vi "REFPROPdll.vi"(8 "error in (no error)":errorcluster, 11 "Inputs":T2) -> (0 "error out":errorcluster, 3 "Outputs":T1)   [LabVIEW 2021]
doc: "subroutine REFPROPdll(hFld, hIn, hOut, iUnits, iMass, iFlag, a, b, zm, Output, hUnits, iUCode, x, y, x3, q, ierr, herr, hFld_length, hIn_length, hOut_length, hUnits_length, herr_length)\n\nCalculate the properties identified in the hOut string for the inputs specified in the hIn string for the fluid or\nmixture given in the hFld string. The unit identifier for the properties should be passed in the iUnits variable (as described below). Compositions can be sent as mole fractions or mass fractions in the zm array depending on the value of iMass.\n\nSeveral items must be considered before using this routine. The most important is the speed of calculations. The original fortran code that called dedicated functions such as TPRHO, TPFLSH, PHFLSH, and so on (mostly given in FLSH_SUB.FOR) and the non-iterative functions such as THERM and TRNPRP requires very little (or none) string comparisons and are quite fast. Multiple string comparisons are made to determine the inputs and outputs the user has selected. Due to the limitation of Fortran in string parsing, this will cause a dramatic increase in the time required to make the calculations, such as two to three times as long as the dedicated functions. Thus the ease of use of this REFPROP subroutine versus the speed of calculation from the older routines must be considered before developing any application.\n\nINPUTS:\nhFld -- Fluid string. See below.\nhIn -- Input string of properties being sent to the routine.\nhOut -- Various flags are available to gain access to all other features of the REFPROP program.\niUnits -- The unit system to be used for the input and output properties (such as SI, English, etc.) See the details much further below for a complete description of the iUnits input value. NOTE: A mass based value for iUnits does not imply that the input and output compositions are on a mass basis, this is specified with the iMass variable.\niMass -- Specifies if the input composition is mole or mass based.\n0 Input compositions given in mole fractions, quality on a molar basis.\n1 Input compositions given in mass fractions, quality on a mass basis. For two-phase states, the values in x and will be returned on a mass basis if iMass=1. NOTE: If the fluid string sent to this routine contains the word “mass” at the end (and thus contains the composition as well as the names of the fluids), this will have preference over the value of iMass when converting those compositions from a mass to a molar basis.\niFlag -- Flag to specify if the routine SATSPLN should be called (where a value of 1 activates the call). (Eventually this variable may be used to send multiple flags combined in this flag)\na -- First input property as specified in the hIn variable\nb -- Second input property as specified in the hIn variable\nzm -- Composition on a mole or mass basis depending on the value sent in iMass (array of size ncmax=20).\n\nOUTPUTS:\nOutput -- Array of properties specified by the hOut string (array of size 200 dimensioned as double precision). The number -9999970 will be returned when errors occur, and the number -9999990 will be returned when nothing was calculated. Read the comments in the ALLPROPS routine to fully understand the contents of this array.\nhUnits -- The units for the first property in the Output array. Strings such as a fluid name may also be passed back in this position. To obtain the units for all of the properties sent to the string, call the ALLPROPS routine instead.\niUCode -- Unit code that represents the units of the first property in the Output array. See below for further details.\nx -- Composition of the liquid phase (array of mole fractions of size 20) for two-phase states on a mole or mass basis depending on the value of iMass.\ny -- Composition of the vapor phase (array of mole fractions of size 20) for two-phase states on a mole or mass basis depending on the value of iMass.\nx3 -- Reserved for returning the composition of a second liquid phase for LLE or VLLE.\nq -- Vapor quality on a mole or mass basis depending on the value of iMass. (See subroutine ABFLSH for the definitions of values returned for this variable). To obtain the molar quality regardless of iMass, send “qmole” as an input in hIn, and vice-versa for “qmass”.\nierr -- Error flag\nherr -- Error string (character*255)\nhFld_length -- length of variable hFld (default: 10000)\nhIn_length -- length of variable hIn (default: 255)\nhOut_length -- length of variable hOut (default: 255)\nhUnits_length -- length of variable hUnits (default: 255)\nherr_length -- length of variable herr (default: 255)"
uses:
  REFPROP.dll
panel:
  # "REFPROP-REFPROPdll.vi"
  # "void REFPROPdll(char *hFld, char *hIn, char *hOut, int *iUnits, int *iMass, int *iFlag, double *a, double *b, double *z/* 20 */, double *Output/* 200 */, char *hUnits, int *iUCode, double *x/* 20 */, double *y/* 20 */, double *x3/* 20 */, double *q, int *ierr, char *herr, int hFld_length/* 10000 */, int hIn_length/* 255 */, int hOut_length/* 255 */, int hUnits_length/* 255 */, int herr_length/* 255 */);"
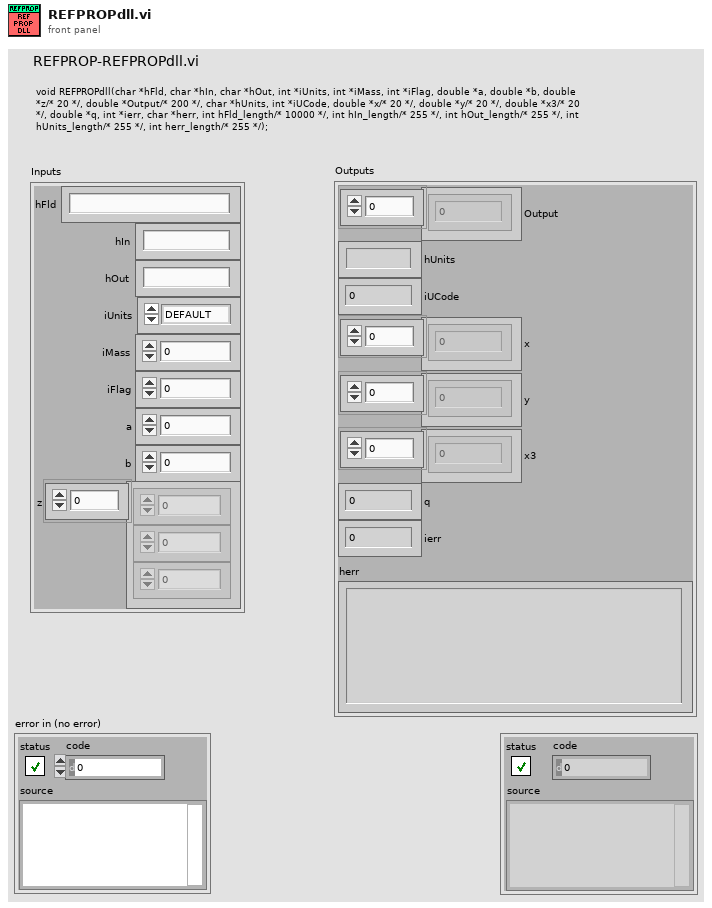
[diagram p1: front panel]
types:
  T1 = cluster{"Output":dbl[], "hUnits":string, "iUCode":i32, "x":dbl[], "y":dbl[], "x3":dbl[], "q":dbl, "ierr":i32, "herr":string}
  T2 = cluster{"hFld":string, "hIn":string, "hOut":string, "iUnits":enum32{"DEFAULT", "MOLE SI", "MASS SI", "SI WITH C"}, "iMass":i32, "iFlag":i32, "a":dbl, "b":dbl, "z":dbl[]}
  T3 = enum32{"DEFAULT", "MOLE SI", "MASS SI", "SI WITH C"}
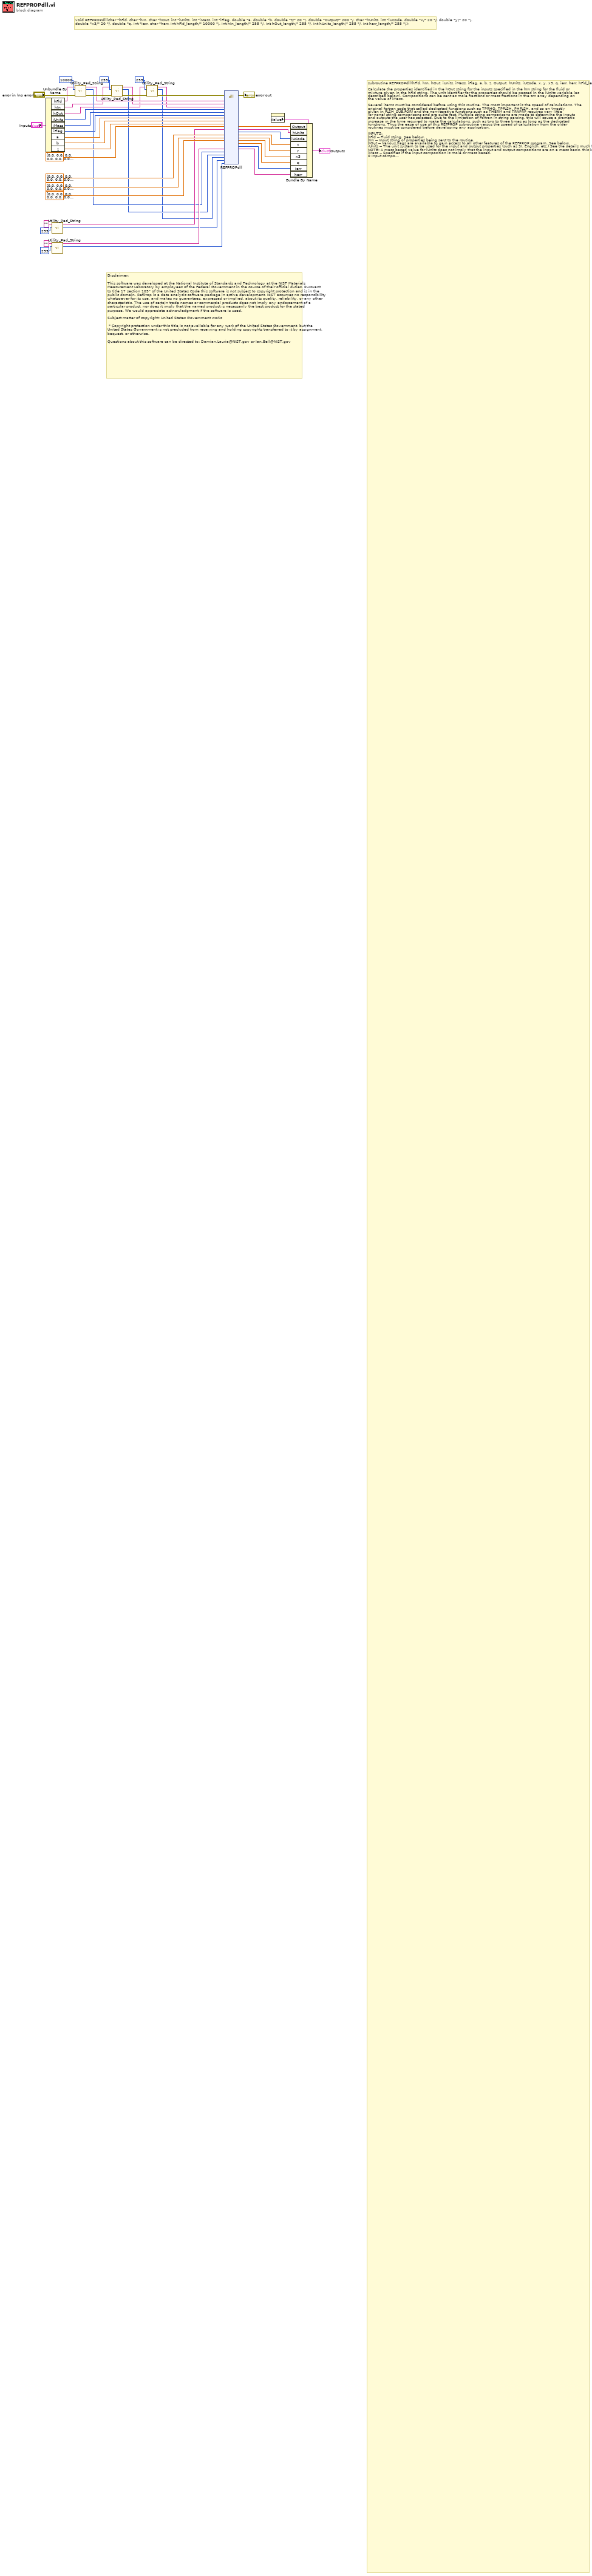
[diagram p0: block diagram]
diagram:
  # "void REFPROPdll(char *hFld, char *hIn, char *hOut, int *iUnits, int *iMass, int *iFlag, double *a, double *b, double *z/* 20 */, double *Output/* 200 */, char *hUnits, int *iUCode, double *x/* 20 */, double *y/* 20 */, double *x3/* 20 */, double *q, int *ierr, char *herr, int hFld_length/* 10000 */, int hIn_length/* 255 */, int hOut_length/* 255 */, int hUnits_length/* 255 */, int herr_length/* 255 */);"
  # "Disclaimer:\n\nThis software was developed at the National Institute of Standards and Technology at the NIST Materials Measurement Laboratory by employees of the Federal Government in the course of their official duties. Pursuant to title 17 section 105* of the United States Code this software is not subject to copyright protection and is in the public domain. RefProp is a data analysis software package in active development. NIST assumes no responsibility whatsoever for its use, and makes no guarantees, expressed or implied, about its quality, reliability, or any other characteristic. The use of certain trade names or commercial products does not imply any endorsement of a particular product, nor does it imply that the named product is necessarily the best product for the stated purpose. We would appreciate acknowledgment if the software is used.\n \nSubject matter of copyright: United States Government works\n  \n * Copyright protection under this title is not available for any work of the United States Government, but the United States Government is not precluded from receiving and holding copyrights transferred to it by assignment, bequest, or otherwise.\n\nQuestions about this software can be directed to: Damian.Lauria@NIST.gov or Ian.Bell@NIST.gov"
  # "subroutine REFPROPdll(hFld, hIn, hOut, iUnits, iMass, iFlag, a, b, z, Output, hUnits, iUCode, x, y, x3, q, ierr, herr, hFld_length, hIn_length, hOut_length, hUnits_length, herr_length)\n\nCalculate the properties identified in the hOut string for the inputs specified in the hIn string for the fluid or\nmixture given in the hFld string. The unit identifier for the properties should be passed in the iUnits variable (as\ndescribed below). Compositions can be sent as mole fractions or mass fractions in the zm array depending on\nthe value of iMass.\n\nSeveral items must be considered before using this routine. The most important is the speed of calculations. The\noriginal fortran code that called dedicated functions such as TPRHO, TPFLSH, PHFLSH, and so on (mostly\ngiven in FLSH_SUB.FOR) and the non-iterative functions such as THERM and TRNPRP requires very little\n(or none) string comparisons and are quite fast. Multiple string comparisons are made to determine the inputs\nand outputs the user has selected. Due to the limitation of Fortran in string parsing, this will cause a dramatic\nincrease in the time required to make the calculations, such as two to three times as long as the dedicated\nfunctions. Thus the ease of use of this REFPROP subroutine versus the speed of calculation from the older\nroutines must be considered before developing any application.\n\nINPUTS:\nhFld -- Fluid string. See below.\nhIn -- Input string of properties being sent to the routine.\nhOut -- Various flags are available to gain access to all other features of the REFPROP program. See below.\niUnits -- The unit system to be used for the input and output properties (such as SI, English, etc.) See the details much further below for a complete description of the iUnits input value. NOTE: A mass based value for iUnits does not imply that the input and output compositions are on a mass basis, this is specified with the iMass variable.\niMass -- Specifies if the input composition is mole or mass based.\n0 Input compositions given in mole fractions, quality on a molar basis.\n1 Input compositions given in mass fractions, quality on a mass basis. For two-phase states, the values in x and\nwill be returned on a mass basis if iMass=1. NOTE: If the fluid string sent to this routine contains the word \n“mass” at the end (and thus contains the composition as well as the names of the fluids), this will have\n preference over the value of iMass when converting those compositions from a mass to a molar basis.\niFlag -- Flag to specify if the routine SATSPLN should be called (where a value of 1 activates the call). (Eventually this variable may be used to send multiple flags combined in this flag)\na -- First input property as specified in the hIn variable\nb -- Second input property as specified in the hIn variable\nzm -- Composition on a mole or mass basis depending on the value sent in iMass (array of size ncmax=20).\n\nOUTPUTS:\nOutput -- Array of properties specified by the hOut string (array of size 200 dimensioned as double precision). The number -9999970 will be returned when errors occur, and the number -9999990 will be returned when nothing was calculated. Read the comments in the ALLPROPS routine to fully understand the contents of this array.\nhUnits -- The units for the first property in the Output array. Strings such as a fluid name may also be passed back in this position. To obtain the units for all of the properties sent to the string, call the ALLPROPS routine instead.\niUCode -- Unit code that represents the units of the first property in the Output array. See below for further details.\nx -- Composition of the liquid phase (array of mole fractions of size 20) for two-phase states on a mole or mass basis depending on the value of iMass.\ny -- Composition of the vapor phase (array of mole fractions of size 20) for two-phase states on a mole or mass basis depending on the value of iMass.\nx3 --  Reserved for returning the composition of a second liquid phase for LLE or VLLE.\nq -- Vapor quality on a mole or mass basis depending on the value of iMass. (See subroutine ABFLSH for the definitions of values returned for this variable). To obtain the molar quality regardless of iMass, send “qmole” as an input in hIn, and vice-versa for “qmass”.\nierr -- Error flag\nherr -- Error string (character*255)\nhFld_length -- length of variable hFld (default: 10000)\nhIn_length -- length of variable hIn (default: 255)\nhOut_length -- length of variable hOut (default: 255)\nhUnits_length -- length of variable hUnits (default: 255)\nherr_length -- length of variable herr (default: 255)\n\nInformation on hFld\nFor a pure fluid, hfld contains the name of the fluid file (with a path if needed).\nFor a mixture, it contains the names of the constituents in the mixture separated by semicolons or asterisks.\nOnce the routine has been called with hFld set to the desired fluids, a space can be sent for all other calls that\nuse the same fluid(s). For a predefined mixture, the extension “.mix” must be included. If the composition is\nincluded in the hFld variable, or if a predefined mixture is selected, the composition will be returned in the zm\narray (on a molar or mass basis depending on iMass.) That composition (or other compositions) must be sent in\nzm in all subsequent calls to this routine. See subroutines SETFLUIDS and SETMIXTURE further below for\nadditional information and examples.\n\nNote: The speed of the program will be increased (sometimes substantially) if you call this routine only once\nwith the name of the fluid and then never again unless your fluid or mixture changes. If your composition\nchanges, send the new composition in the z array rather then sending a new string in the hfld variable.\n\nExamples:\nhFld='NITROGEN'\nhFld='C:/Program Files (x86)/REFPROP/FLUIDS/R1234YF.FLD'\nhFld='CARBON DIOXIDE'\nhFld='METHANE;ETHANE;PROPANE;BUTANE;ISOBUTANE'\nhFld='METHANE*ETHANE*PROPANE*BUTANE*ISOBUTANE'\nhFld='R134a;0.3; R1234yf;0.3; R1234ze(Z);0.4'\nhFld='CO2;0.2 * isobutane;0.3 * propadiene;0.5'\nhFld='Nitrogen;Oxygen;Argon|0.4;0.3;0.3'\nhFld='Nitrogen; Oxygen; Argon ~ 0.4; 0.3; 0.3'\nhFld='R410A.MIX'\n\nInformation on hIn\nValid codes are T, P, D, E, H, S, and Q (temperature, pressure, density, energy, enthalpy, entropy, and quality).\nTwo of these should be sent together to identify the contents of the a and b variables. For example, ‘TP’ would\nindicate inputs of temperature and pressure, and ‘TQ’ would indicate inputs of temperature and quality. A value\nof 0 for the quality will return a saturated liquid state, and a value of 1 will return a saturated vapor state. A\nvalue between 0 and 1 will return a two-phase state. Valid inputs are: TP, TD, TE, TH, TS, TQ, PD, PE, PH, PS,\nPQ, DE, DH, DS, DQ, ES, EQ, HS, HQ, SQ (or the inverse of any of these, e.g., QT) (hIn is not case sensitive,\ne.g., ‘TQ’ = ‘tq’). When q is >0 and <1, then the quality uses a molar basis when iMass=0 and a mass basis\nwhen iMass=1. The value of iUnits has no effect on the value of q (as either an input or output). The shortcuts\nTsat and Psat can be used to specify a saturation state for the liquid for a pure fluid. To return, for example, the\nsaturated vapor density, Dvap would be used as an output variable. The order of the properties being sent to the\nroutine in the variables a and b has to be the same as the letters sent to hIn; for example, if hIn is ‘QT’, then a=q\nand b=T.\n\nThe ABFLSH routine is called to determine the phase of the inputs (liquid, vapor, or 2-phase), and then the\nappropriate iterative routine will be called to obtain the independent properties of the equations of state: these\nbeing temperature and density. For subsequent calculations for properties that are in the single phase, use the\ncode TD&, where the symbol & indicates the single phase state. The time required with the use of TD& is\nnegligible compared to that required for the iterative solution called by ABFLSH. However, the properties sent\nto this routine and the calculated outputs are cached to avoid additional iterative calls when the solution has\nalready been determined. Be sure to read the warnings at the top of the ALLPROPS routine for additional\ninformation.\n\nFlags to specify certain phases are listed below, for example, ‘TD>’ would specify an input state in the liquid\nphase but which would normally be two-phase. Those available are:\n\n• **> or **L: When the letter ‘L’ is attached after the two letters that specify the input properties (such as\n‘TP’), the routine will assume that the input properties are in the single phase liquid region, or are within\nthe two-phase area as a metastable state. For example: TP>, PH>, HSL\n\n• **< or **V: The letter ‘V’ (or the sign ‘<’) specifies that the input state for the properties listed in the first\ntwo letters is in the single phase vapor (including metastable states). For example: TP<, PH<, HSV\n• TH< or TH>: Inputs of temperature and enthalpy (or occasionally temperature and internal energy) generally\nhave two valid states. To obtain the root with the higher pressure, use TH> or TE>, and for the lower\npressure use TH< or TE<.\n\n• *MELT: Return properties at the melting point where the input property is specified by the *, for example\nTMELT requires the temperature for the input variable a, PMELT requires the pressure for input variable\na, and so on.\n\n• *SUBL: Return properties at the sublimation point, as described above for the melting point.\n\n• CRIT: Return properties at the critical point (for example, hIn=’CRIT’ and hOut=’S’ would return the\nentropy at Tc and Dc). For a mixture, the critical point defined by the equation of state is only available if\nthe SATSPLN routine has been called, otherwise an estimated value is returned.\n\n• TRIP: Return liquid phase properties at the triple point.\n\n• NBP: Return properties at the normal boiling point.\n\n• DSAT: Return the saturation properties for the input density.\n\n• HSAT, HSAT2: Enthalpy can be doubled valued in the vapor phase for some fluids. In such a situation,\nHSAT2 will return the root with the lower temperature.\n\n• SSAT, SSAT2, SSAT3: Entropy can be doubled or triple valued in the vapor phase for some fluids (see\nbutane for example). In such a situation, SSAT will return the root at the highest temperature, SSAT2 will\nreturn the middle root, and SSAT3 will return the root with the lowest temperature.\n\nVarious flags are available that can be sent to this routine in the variable hIn to gain access to all other features\nof the REFPROP program. These cannot be combined as multiple inputs in hIn:\n\n• FLAGS: Call the FLAGS routine at the bottom of this file to initialize the options available for controlling\ncertain aspects of the REFPROP program. Some of these include caching properties, turning on/off different\ntypes of equations of state (Peng-Robinson, GERG-2008, and AGA-8), the calorie to Joule definition,\nand so on. The flag string (the first input to the FLAGS routine) should be sent in hOut and the flag option\nin iFlag. The output (3rd variable in the routine) is returned in iUCode. See the FLAGS routine for further\ninformation. The variable hFld for the REFPROP routine should be left blank when using this option.\n\n• EOSMIN: Return the property specified in hOut at the minimum temperature allowed in the equation of\nstate. This is generally at the triple point in the liquid phase. Note that an input of P or D will not return the\nobvious minimum (zero), but the pressure and density at the liquid phase triple point (or lower temperature\nlimit for a mixture). For water, the triple point T is still returned, even though lower temperatures are\npossible.\n\n• EOSMAX: Return the maximum temperature, pressure, or density (as specified in hOut) for the equation\nof state. The maximum density of the equation of state does not occur at the maximum pressure and\ntemperature. Only T, P, or D can be returned one at a time to emphasize that properties at Tmax and Pmax\nare not the same as at Tmax and Dmax.\n\n• SETREF: Call the SETREF routine. The reference state (DEF, NBP, IIR, ASH, OTH, OT0, or NA) should\nbe sent in hOut. For the OTH and OT0 options, the values of h0, s0, T0, and P0 should be included in the\nhOut variable, separated by semicolons. For example: hOut='OTH;10.;1.;323.15;101.325'\n\nThis would set the enthalpy to 10 J/mol and the entropy to 1 J/mol-K at 323.15 K and 101.325 kPa. In\nthe GUI is an option for mixtures to set the reference state to either the composition in use or to each pure\nfluid. To set this option through the DLL, a value of either 1 or 2 should be sent to this routine in the\nvariable a. This will set the variable labeled ixflag in subroutione SETREF in the SETUP.FOR file. All\nother options for this command are also explained in the SETUP.FOR file.\n\n• SETREFOFF: Turn off the inputs that were sent in the option above.\n\n• PATH: Call the SETPATH routine with the path given in hFld.\n\n• SATSPLN: Call the SATSPLN routine for the input composition (as described in the SAT_SUB.FOR file).\nThe fluid name or mixture names and the composition must be sent with this command or have already\nbeen setup before this is called. This command is identical to calling this routine with iFlag=1, except that\nit can be issued at any time.\n\nInformation on hOut\nString output is returned in hUnits. Numerical output is returned in Output(1). For flags used to obtain a value\nof a particular fluid in a mixture, the component number should be added after the command, such as NAME(3)\nor FDIR(1). Only one string output can be requested at a time for the following flags, down to the line that\nsays DLL#. Use the ALLPROPS routine to return multiple strings for all the components in the mixture. This\nis done without using the component number, e.g., sending “NAME” to that routine. For numerical values,\nmultiple inputs can be requested here, and must be separated by spaces, commas, semicolons, or bars, but these\nseparators should not be mixed. See subroutine ALLPROPS (which follows this routine) for further information.\n\n• ALTID: Return the alternative fluid whose mixing rules are used when others are not available.\n\n• CAS#: Return the CAS number.\n\n• CHEMFORM: Return the short chemical formula.\n\n• SYNONYM: Return the synonym found on the fifth line in the fluid files.\n\n• FAMILY: Return the family class used for several predictive schemes.\n\n• FLDNAME: Return the fluid file name sent to the SETUP routine.\n\n• HASH: Return the hash number.\n\n• INCHI: Return the INCHI string.\n\n• INCHIKEY: Return the INCHI key.\n\n• LONGNAME: Return the long fluid name given in the 3rd line of the fluid files.\n\n• SAFETY: Return the ASHRAE 34 classification.\n\n• NAME: Return the fluid short name.\n\n• NCOMP: Return the number of components.\n\n• UNNUMBER: Return the UN number.\n\n• EOSDOI: Return the DOI of the equation of state.\n\n• VISDOI: Return the DOI of the viscosity correlation.\n\n• TCXDOI: Return the DOI of the thermal conductivity correlation.\n\n• STNDOI: Return the DOI of the surface tension equation.\n\n• DIEDOI: Return the DOI of the dielectic constant correlation.\n\n• MLTDOI: Return the DOI of the melting line equation.\n\n• SBLDOI: Return the DOI of the sublimation line equation.\n\n• REFSTATE: Return the reference state in use (NBP, IIR, ASH, OTH, etc.)\n\n• GWP: Return the global warming potential (found in the fluid file header).\n\n• ODP: Return the ozone depletion potential (found in the fluid file header).\n\n• FDIR: Return the location (directory) of the fluid file. The directory is returned in both the hUnits string\nand in herr if no other error occurred (paths that are more than 50 characters long are truncated in hUnits).\nAn error code of -999 will also be returned that can be used to check if herr is the path and not another\nerror message. For mixtures, send FDIR(2), etc., to get the path of the second fluid and so on.\n\n• UNITSTRING: Return the units of the property (e.g., K, psia, kg/m^3, J/mol, etc.) identified in hIn for\nthe unit system defined in hFld (e.g., SI, E, etc.). The input values for hIn are the labels described in the\nALLPROPS routine. For example, ‘D2DDP2’ would return ‘(kg/m^3)/MPa^2’ for ‘SI’ inputs.\n\n• UNITNUMB: Return in iUCode the integer value associated with a particular set of units defined in hFld\n(SI, E, etc.). This integer value can then be used in subsequent calls for the iUnits variable.\n\n• UNITS: Perform both operations in UNITSTRING and UNITNUMB.\n\n• UNITCONV: Convert the property contained in the variable a from units given in hFLD to units given\nin hIn. The unit strings are given much further below. When converting from mole to mass units (or\nvice versa), the molar mass must be sent in the variable b. The type of property (as specified in the\nCONVUNITS subroutine) must be appended to the string in hOut, for example, hOut=’UNITCONV_T’\nor hOut=’UNITCONV_D’\n\n• UNITUSER, UNITUSER2: Set a predefined set of units based on the user’s need. Two different sets\ncan be assigned depending on the input sent to the routine. The variable hIn contains the numbers that\nare specified by the enumerations in the CONSTS.INC file, separated by semicolons. For example,\nhIn=‘0;157;0;0;0;403;0;0;0;0’ would set the pressure to use units of atm and the speed of sound to use\nunits of km/h. The numbers are listed in the order of T, P, D, H, S, W, I, E, K, and N. (temperature,\npressure, density, enthalpy, entropy, speed of sound, kinematic viscosity, viscosity, thermal conductivity,\nand surface tension). Because the enumerations might change, it is best to build this string with the\nenumerations listed in the CONSTS.INC file rather than hard coding the numbers as shown above.\n• DLL#: Return the version number of the DLL in iUCode and the string value in hUnits.\n\n• PHASE: Return the phase of the state for the input fluids and properties. See subroutine PHASE for a\nlisting of all possibilities. The output is sent back in the hUnits variable. No other command can be sent\nwith this one since hUnits is not an array.\n\n• FULLCHEMFORM: Return the long chemical formula.\n\n• HEATINGVALUE: Return the upper heating value.\n\n• LIQUIDFLUIDSTRING: Return a string that contains the fluid names and compositions for the liquid\nphase of a two-phase state.\n\n• VAPORFLUIDSTRING: Likewise for the vapor phase. For example, “R32;R125|0.25;0.75”. The string is\npassed back in hUnits.\n\n• Q: Return the quality on a molar or mass basis depending on the value of iMass. This option is not\nrecommended, rather use QMOLE or QMASS to eliminate the use of the wrong unit system.\n\n• QMOLE: Return the molar quality for 2-phase states.\n\n• QMASS: Return the mass quality for 2-phase states.\n\n• XMASS: Return the mass compositions in the Output array as with the X command. See comment one line\nup.\n\n• XLIQ: Return the mass or molar liquid compositions (depending on the value of iMass) for 2-phase states.\n\n• XVAP: Return the mass or molar vapor compositions (depending on the value of iMass) for 2-phase states.\n\n• XMOLELIQ: Return the liquid compositions for 2-phase states on a mole basis regardless of the iMass\nvariable.\n\n• XMOLEVAP: Return the vapor compositions for 2-phase states on a mole basis regardless of the iMass\nvariable.\n\n• XMASSLIQ: Return the liquid compositions for 2-phase states on a mass basis regardless of the iMass\nvariable.\n\n• XMASSVAP: Return the vapor compositions for 2-phase states on a mass basis regardless of the iMass\nvariable.\n\n• *LIQ: (where * is T, P, D, etc.) Return the liquid saturation properties for the property listed as the first\nletter. This is only valid for saturation states or 2-phase states.\n\n• *VAP: (where * is T, P, D, etc.) Return the vapor saturation properties for the property listed as the first\nletter. This is only valid for saturation states or 2-phase states.\n\n• FIJMIX: Return the mixing parameters in the first six slots of the variable Output for the binary mixture\nidentified by the values in the a and b variables (i.e., integer values are sent in double precision variables). The mixing rule is returned in the hUnits string.\n\nInformation on iUnits\nMultiple unit systems are available for use in property values, such as the SI system, English system, mixed sets,\nand so forth. Each set is identified with an enumerated value, which is sent as an input code in iUnits.\n\n<FORTRAN ONLY> \n\nThe enumerated value for the different unit systems are listed below and in the CONSTS.\nINC file, which can be included in your FORTRAN program, as such:\ninclude 'CONSTS.INC'\n\nWarning: Do NOT include any other INC file in your programs\nThe enumerated values for the unit systems are given by the parameters\n• iUnitsMolSI\n• iUnitsSI\n• . . .\n\n</FORTRAN ONLY>\n\nIn all environments other than FORTRAN, the iUnits variable should be retrieved from the GETENUMdll()\nfunction with a call like:\n\nGETENUMdll(0,'MOLAR BASE SI',iEnum,ierr,herr)\n\nWarning: The integer values for iUnits given below should NEVER be used directly, you should always retrieve\nthe enumerated value from GETENUMdll(). This is to allow the developers of REFPROP flexibility\nin the future.\n\nThe unit systems used in REFPROP are as follows:\n\n                                            DEFAULT                  MOLE SI              MASS SI               SI WITH C\niUnits --->                          0                                1                           2                           3\nTemperature                      K                                K                          K                           C\nPressure                              KPa                           MPa                    MPa                      MPa\nDensity                               mol/dm^3               mol/dm^3         kg/m^3                kg/m^3\nEnthalpy                             J/mol                         J/mol                  J/g                         J/g\nEntropy                             (J/mol)/K                  (J/mol)/K            (J/g)/K                  (J/g)/K\nSpeed                                 m/s                            m/s                    m/s                       m/s\nKinematic vis.                   cm^2/s                      cm^2/s             cm^2/s                cm^2/s\nViscosity                            uPa-s                          uPa-s                uPa-s                    uPa-s\nThermal cond.                  W/(m-K)                    mW/(m-K)       mW/(m-K)          mW/(m-K)\nSurface tension                 N/m                           mN/m              mN/m                  mN/m\nMolar Mass                        g/mol                        g/mol                g/mol                   g/mol\n\n\n                                            MOLAR MASS\n                                            BASE SI                       BASE SI              ENGLISH              MOLAR ENGLISH\niUnits --->                          100                             101                     5                            6\nTemperature                      K                                 K                        F                            F\nPressure                              Pa                               Pa                      psia                       psia\nDensity                                mol/m^3                  kg/m^3            lbm/ft^3              lbmol/ft^3\nEnthalpy                              J/mol                         J/kg                   Btu/lbm               Btu/lbmol\nEntropy                              (J/mol)/K                   (J/kg)/K            (Btu/lbm)/R        (Btu/lbmol)/R\nSpeed                                  m/s                             m/s                   ft/s                       ft/s\nKinematic vis.                    m^2/s                         m^2/s              ft^2/s                  ft^2/s\nViscosity                             Pa-s                             Pa-s                  lbm/(ft-s)           lbm/(ft-s)\nThermal cond.                   W/(m-K)                    W/(m-K)           Btu/(h-ft-R)       Btu/(h-ft-R)\nSurface tension                  N/m                            N/m                  lbf/ft                    lbf/ft\nMolar Mass                         kg/mol                        kg/mol            lbm/lbmol          lbm/lbmol\n\n                                             MKS                             CGS                   MIXED                MEUNITS\niUnits --->                           7                                   8                        9                         10\nTemperature                       K                                  K                        K                         C\nPressure                               kPa                              MPa                  psia                     bar\nDensity                                 kg/m^3                      g/cm^3           g/cm^3              g/cm^3\nEnthalpy                               J/g                              J/g                     J/g                       J/g\nEntropy                                (J/g)/K                       (J/g)/K              (J/g)/K                 (J/g)/K\nSpeed                                   m/s                            cm/s                  m/s                     cm/s\nKinematic vis.                     cm^2/s                      cm^2/s             cm^2/s              cm^2/s\nViscosity                              uPa-s                         uPa-s                 uPa-s                  cpoise   \nThermal cond.                   W/(m-K)                     mW/(m-K)       mW/(m-K)         mW/(m-K)\nSurface tension                  mN/m                        dyne/cm           mN/m               mN/m\nMolar Mass                         g/mol                         g/mol                g/mol                g/mol\n\n                                             USER (can be changed by calling the REFPROP subroutine)\niUnits --->                           11\nTemperature                       C\nPressure                               psig\nDensity                                kg/m^3\nEnthalpy                              J/g\nEntropy                              (J/g)/K\nSpeed                                  m/s\nKinematic vis.                    cm^2/s\nViscosity                             mPa-s\nThermal cond.                   W/(m-K)\nSurface tension                  N/m\nMolar Mass                         g/mol\n\nInformation on iUCode output\nThe iUCode variable uses a four digit code that specifies the units of the property:\n\n• Left digit : Energy unit in J/mol or kJ/kg\n\n• Left middle digit : Density unit in mol/dm^3 or kg/m^3\n\n• Right middle digit : Pressure unit in kPa\n\n• Right digit : Temperature unit in K\n\nEach digit indicates the power of the unit, for example, a value of 2 for the temperature digit corresponding to\nK^2. Values from 6 to 9 specify a negative power digit, for example, a value of 8 would be 1/kPa^2.\n\nThe following values give other examples:\n\n1000       J/mol\n0100      mol/dm^3\n0010      kPa\n0001      K\n0000      - (a value of zero assumes a dimensionless unit)\n9000      1/(J/mol)\n0910      kPa/(mol/dm^3)\n0190      (mol/dm^3)/kPa\n8765      K^5/[(J/mol)^2*(mol/dm^3)^3*kPa^4]\n2082      (J/mol)^2*K^2/kPa^2\n0830      kPa^3/(mol/dm^3)^2\n9281      (mol/dm^3)^2*K/[(J/mol)*kPa^2]\n8139      (mol/dm^3)*kPa^3/[(J/mol)^2*K]\n2288      (J/mol)^2*(mol/dm^3)^2/[kPa^2*K^2]\n1764      (J/mol)*K^4/[(mol/dm^3)^3*kPa^4]\n4857      (J/mol)^4*kPa^5/[(mol/dm^3)^2*K^3]\n2730      (J/mol)^2*kPa^3/(mol/dm^3)^3\n6666      1/[(J/mol)^4*(mol/dm^3)^4*kPa^4*K^4]\n\nNegative values represent special units not built on these four property types:\n\nProperty                               Parameter           Current Value (but subject to change)\nSpeed of sound                   iUTypeW             -9\nViscosity                               iUTypeU              -10\nThermal conductivity         iUTypeK              -11\nSurface tension                   iUTypeN              -12\nQuality                                  iUType0               -13\nMolar mass                          iUTypeM             -14\nKinematic viscosity             iUTypeI                -17\nMass flux                              iUTypeF               -27\nHeating value (volume)     iUTypeG              -37\nDipole moment                   iUTypeB              -38\n\nThe dimension statements for these variables are (in Fortran):\n\nparameter (ncmax=20) !Maximum number of components in the mixture\n\nparameter (iPropMax=200) !Number of output properties available in ALLPROPS.\n\ncharacter*255 hFld,hIn,hOut,hUnits,herr !hFld, hIn, and hOut can actually be of any length.\n\ninteger iUnits,iMass,iFlag,ierr,iUCode !Note: as integer*4\n\ndouble precision a,b,q,Output(iPropMax),zm(ncmax),x(ncmax),y(ncmax),x3(ncmax)"
  n1 = Unbundle By Name("Inputs") -> ("hFld"=w9:string, "hIn"=w6:string, "hOut"=w3:string, "iUnits"=w25:T3, "iMass"=w38:i32, "iFlag"=w37:i32, "a"=w36:dbl, "b"=w35:dbl, "z"=w34:dbl[])
  n2 = call "Utility_Pad_String.vi"("Target Length"=255, "String in"="") -> ("Length out"=w17:i32, "result string"=w18:string)  [unwired: 7 in, 1 out]
  n3 = call "Utility_Pad_String.vi"("Target Length"=255, "String in"="") -> ("Length out"=w19:i32, "result string"=w20:string)  [unwired: 7 in, 1 out]
  n4 = call "Utility_Pad_String.vi"("error in (no error)"="error in (no error)", "Target Length"=10000, "String in"=w9) -> ("error out"=w13:errorcluster, "Length out"=w7:i32, "result string"=w8:string)  [unwired: 6 in]
  n5 = call "Utility_Pad_String.vi"("error in (no error)"=w13, "Target Length"=255, "String in"=w6) -> ("error out"=w12:errorcluster, "Length out"=w4:i32, "result string"=w5:string)  [unwired: 6 in]
  n6 = call "Utility_Pad_String.vi"("error in (no error)"=w12, "Target Length"=255, "String in"=w3) -> ("error out"=w11:errorcluster, "Length out"=w1:i32, "result string"=w2:string)  [unwired: 6 in]
  n7 = dll-call lib="C:/Users/lauria/OneDrive - NIST/LabVIEW Projects/7 REFPROP/REFPROP-wrappers-master/REFPROP-wrappers-master/wrappers/LabVIEW/REFPROP/REFPROP.*" fn="REFPROPdll"(error in=w11, "hFld"=w8, "hIn"=w5, "hOut"=w2, "iUnits"=w25, "iMass"=w38, "iFlag"=w37, "a"=w36, "b"=w35, "z"=w34, "Output"=dbl[] [0.0, 0.0, 0.0, 0.0, 0.0, 0.0, 0.0, 0.0, 0.0, 0.0, 0.0, 0.0, 0.0, 0.0, 0.0, 0.0, 0.0, 0.0, 0.0, 0.0, 0.0, 0.0, 0.0, 0.0, 0.0, 0.0, 0.0, 0.0, 0.0, 0.0, 0.0, 0.0, 0.0, 0.0, 0.0, 0.0, 0.0, 0.0, 0.0, 0.0, 0.0, 0.0, 0.0, 0.0, 0.0, 0.0, 0.0, 0.0, 0.0, 0.0, 0.0, 0.0, 0.0, 0.0, 0.0, 0.0, 0.0, 0.0, 0.0, 0.0, 0.0, 0.0, 0.0, 0.0, 0.0, 0.0, 0.0, 0.0, 0.0, 0.0, 0.0, 0.0, 0.0, 0.0, 0.0, 0.0, 0.0, 0.0, 0.0, 0.0, 0.0, 0.0, 0.0, 0.0, 0.0, 0.0, 0.0, 0.0, 0.0, 0.0, 0.0, 0.0, 0.0, 0.0, 0.0, 0.0, 0.0, 0.0, 0.0, 0.0, 0.0, 0.0, 0.0, 0.0, 0.0, 0.0, 0.0, 0.0, 0.0, 0.0, 0.0, 0.0, 0.0, 0.0, 0.0, 0.0, 0.0, 0.0, 0.0, 0.0, 0.0, 0.0, 0.0, 0.0, 0.0, 0.0, 0.0, 0.0, 0.0, 0.0, 0.0, 0.0, 0.0, 0.0, 0.0, 0.0, 0.0, 0.0, 0.0, 0.0, 0.0, 0.0, 0.0, 0.0, 0.0, 0.0, 0.0, 0.0, 0.0, 0.0, 0.0, 0.0, 0.0, 0.0, 0.0, 0.0, 0.0, 0.0, 0.0, 0.0, 0.0, 0.0, 0.0, 0.0, 0.0, 0.0, 0.0, 0.0, 0.0, 0.0, 0.0, 0.0, 0.0, 0.0, 0.0, 0.0, 0.0, 0.0, 0.0, 0.0, 0.0, 0.0, 0.0, 0.0, 0.0, 0.0, 0.0, 0.0, 0.0, 0.0, 0.0, 0.0, 0.0, 0.0, 0.0, 0.0, 0.0, 0.0, 0.0, 0.0], "hUnits"=w18, "x"=dbl[] [0.0, 0.0, 0.0, 0.0, 0.0, 0.0, 0.0, 0.0, 0.0, 0.0, 0.0, 0.0, 0.0, 0.0, 0.0, 0.0, 0.0, 0.0, 0.0, 0.0], "y"=dbl[] [0.0, 0.0, 0.0, 0.0, 0.0, 0.0, 0.0, 0.0, 0.0, 0.0, 0.0, 0.0, 0.0, 0.0, 0.0, 0.0, 0.0, 0.0, 0.0, 0.0], "x3"=dbl[] [0.0, 0.0, 0.0, 0.0, 0.0, 0.0, 0.0, 0.0, 0.0, 0.0, 0.0, 0.0, 0.0, 0.0, 0.0, 0.0, 0.0, 0.0, 0.0, 0.0], "herr"=w20, "hFld_length"=w7, "hIn_length"=w4, "hOut_length"=w1, "hUnits_length"=w17, "herr_length"=w19) -> (error out=→"error out":errorcluster, "Output"=w39:dbl[], "hUnits"=w45:string, "iUCode"=w44:i32, "x"=w43:dbl[], "y"=w42:dbl[], "x3"=w41:dbl[], "q"=w29:dbl, "ierr"=w28:i32, "herr"=w27:string)  [unwired: 20 in, 1 out]
  n8 = property on="Outputs" class="Clust (strict)"() -> ("Value"=w47:T1)  [unwired: 2 in, 2 out]
  n9 = Bundle By Name(cluster=w47, "Output"=w39, "hUnits"=w45, "iUCode"=w44, "x"=w43, "y"=w42, "x3"=w41, "q"=w29, "ierr"=w28, "herr"=w27) -> (→"Outputs":T1)
